vi "FirstHallSensorSimulator.vi"() -> ()   [LabVIEW 2014]
uses:
  <vilib>/DAQmx/create/channels.llb/DAQmx Create Channel (AO-Voltage-Basic).vi
  <vilib>/DAQmx/configure/timing.llb/DAQmx Timing (Sample Clock).vi
panel:
  out "Waveform":waveform(dbl)(graph)
  out "Actual RPM":dbl=0.1
  in  "Set RPM":dbl(knob)=0.1 scale=60.0..2000.0
  in  "physical channels":tag="Dev1/ao0"
  in  "AO Rate":dbl=1000.0 format="%0.2f"
  in  "stop":bool
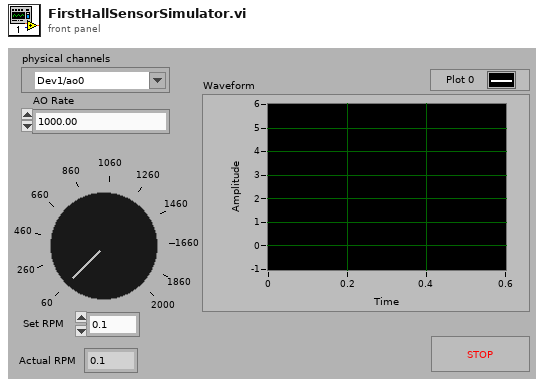
[diagram p1: front panel]
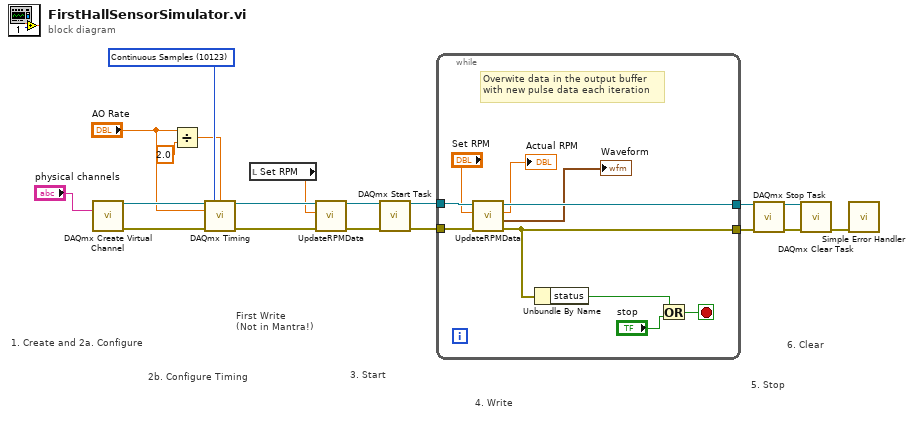
[diagram p0: block diagram]
diagram:
  w15 = 10123 items=["Finite Samples"=10178, "Continuous Samples"=10123] ("sample mode")
  # "6. Clear"
  # "5. Stop"
  # "4. Write"
  # "3. Start"
  # "First Write\n(Not in Mantra!)"
  # "2b. Configure Timing"
  # "1. Create and 2a. Configure"
  n1 = call-poly <vilib>:"DAQmx Create Virtual Channel.vi"("physical channels"="physical channels") -> ("task out"=w14:refnum<k21>, "error out"=w13:errorcluster)  [unwired: 13 in]
  n2 = Divide(x="AO Rate", y=2.0) -> (x/y=w5:dbl)
  n3 = call-poly <vilib>:"DAQmx Timing.vi"("task/channels in"=w14, "sample mode"=w15, "samples per channel"=w5, "rate"="AO Rate", "error in"=w13) -> ("task out"=w12:refnum<k21>, "error out"=w10:errorcluster)  [unwired: 9 in]
  n4 = local read "Set RPM"() -> (w8:dbl)
  n5 = call "UpdateRPMData.vi"("error in (no error)"=w10, "RPM"=w8, "Refnum in"=w12) -> ("error out"=w9:errorcluster, "Refnum out"=w11:refnum<k21>)  [unwired: 3 in, 2 out]
  n6 = call <vilib>:"DAQmx Start Task.vi"("task/channels in"=w11, "error in"=w9) -> ("task out"=w19:refnum<k21>, "error out"=w18:errorcluster)  [unwired: 12 in]
  n7 = while {
    tunnel: w19 -> [w26]
    tunnel: w18 -> [w25]
    tunnel: [w23] -> w3
    tunnel: [w24] -> w4
    stop <- w27 stop-if-true
    # "Overwite data in the output buffer\nwith new pulse data each iteration"
    n8 = call "UpdateRPMData.vi"("error in (no error)"=w25, "RPM"="Set RPM", "Refnum in"=w26) -> ("error out"=w23:errorcluster, "Waveform"=→"Waveform":waveform(dbl), "RPM out"=→"Actual RPM":dbl, "Refnum out"=w24:refnum<k21>)  [unwired: 3 in]
    n9 = Unbundle By Name(w23) -> ("status"=w29:bool)
    n10 = Or(x=w29, y="stop") -> (x .or. y?=w27:bool)
  }
  n11 = call <vilib>:"DAQmx Stop Task.vi"("task/channels in"=w4, "error in"=w3) -> ("task out"=w1:refnum<k21>, "error out"=w2:errorcluster)  [unwired: 12 in]
  n12 = call <vilib>:"DAQmx Clear Task.vi"("task in"=w1, "error in"=w2) -> ("error out"=w17:errorcluster)  [unwired: 13 in]
  n13 = call <vilib>:"Simple Error Handler.vi"("error in (no error)"=w17) -> ()  [unwired: 4 in, 5 out]
